vi "FCI Bin Test_102.vi"(8 "Error In":errorcluster, 9 "Calibration Image in":T1, 10 "Measurement Values array in":dbl[](array[numeric]), 11 "Image In":T1) -> (0 "Error Out":errorcluster, 1 "Measurement Values array out":dbl[](array[numeric]), 2 "102 Results":T2, 3 "Image Out":T1(plugin-control))   [LabVIEW 2019, in "Algorithm.lvclass"]
uses:
  FrameworkOverrides/Algorithm.lvclass
  <vilib>/vision/Image Controls.llb/IMAQ Image.ctl
panel:
  out "Algo Execution Time":u64
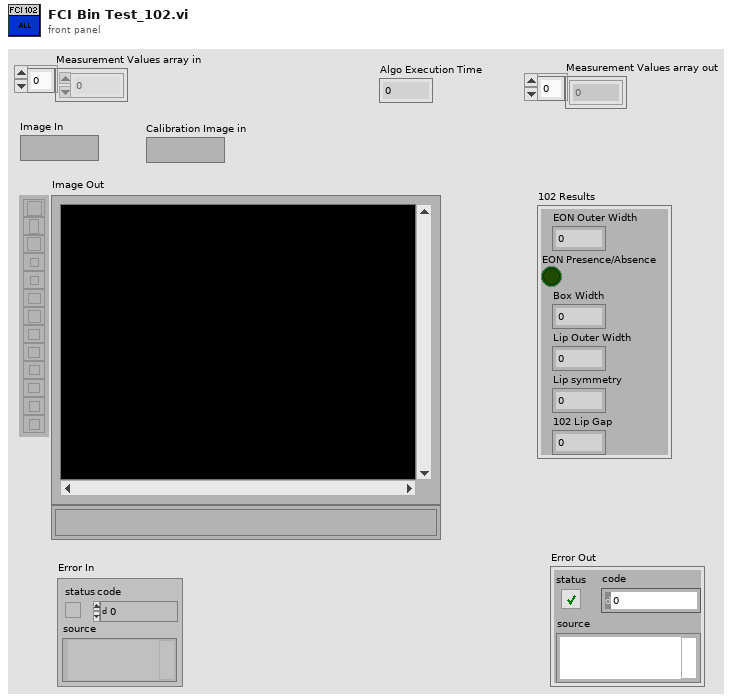
[diagram p1: front panel]
types:
  T1 = typedef "IMAQ Image.ctl" = refnum<image>
  T2 = cluster{"EON Outer Width":sgl, "EON Presence/Absence":bool, "Box Width":sgl, "Lip Outer Width":sgl, "Lip symmetry":dbl, "102 Lip Gap":sgl}
  T3 = cluster{"Box Width M ROI":cluster{"Left":dbl, "Top":dbl, "Right":dbl, "Bottom":dbl, "Angle":dbl}, "EON Outer Width M ROI":cluster{"Left":dbl, "Top":dbl, "Right":dbl, "Bottom":dbl, "Angle":dbl}, "Lip Outer Width M ROI":cluster{"Left":dbl, "Top":dbl, "Right":dbl, "Bottom":dbl, "Angle":dbl}, "102 Lip Gap M ROI":cluster{"Left":dbl, "Top":dbl, "Right":dbl, "Bottom":dbl, "Angle":dbl}}
  T4 = cluster{"Left":dbl, "Top":dbl, "Right":dbl, "Bottom":dbl, "Angle":dbl}
  T5 = typedef "Image Type" = u32
  T6 = cluster{"Centre X":dbl, "Centre Y":dbl, "Angle":dbl}
  T7 = cluster{"First Edges":cluster{"X":sgl, "Y":sgl}[], "Last Edges":cluster{"X":sgl, "Y":sgl}[]}
  T8 = cluster{cluster{"X":sgl, "Y":sgl}, cluster{"X":sgl, "Y":sgl}}[]
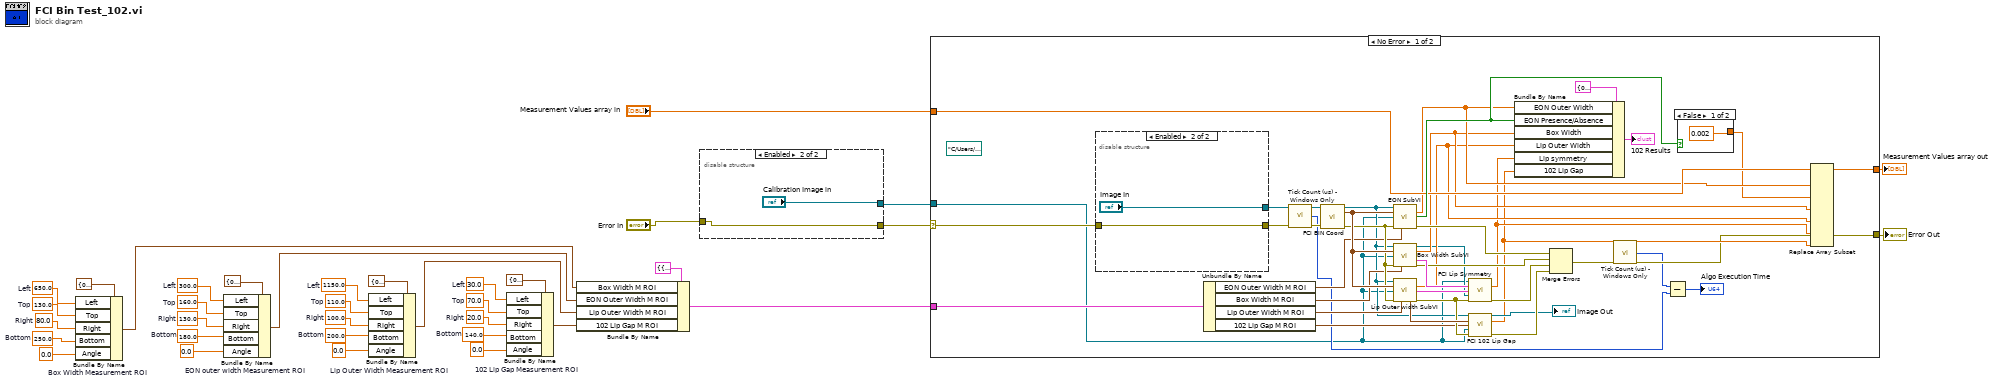
[diagram p0: block diagram]
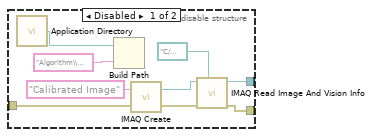
[diagram p2: hidden frame]
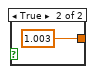
[diagram p3: hidden frame]
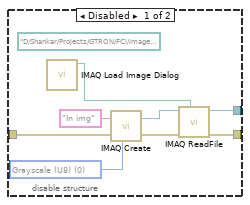
[diagram p4: hidden frame]
diagram:
  w27 = 140.0  # Bottom
  w28 = 20.0  # Right
  w29 = 70.0  # Top
  w30 = 30.0  # Left
  w21 = 200.0  # Bottom
  w20 = 100.0  # Right
  w19 = 110.0  # Top
  w18 = 1150.0  # Left
  w16 = 180.0  # Bottom
  w15 = 130.0  # Right
  w14 = 160.0  # Top
  w13 = 300.0  # Left
  w10 = 250.0  # Bottom
  w9 = 80.0  # Right
  w8 = 130.0  # Top
  w7 = 650.0  # Left
  n1 = Bundle By Name "Box Width Measurement ROI"(cluster=T4 {"Left"=0.0, "Top"=0.0, "Right"=0.0, "Bottom"=0.0, "Angle"=0.0} ("input cluster"), "Left"=w7, "Top"=w8, "Right"=w9, "Bottom"=w10, "Angle"=0.0) -> (w32:T4)
  n2 = Bundle By Name "EON outer width Measurement ROI"(cluster=T4 {"Left"=0.0, "Top"=0.0, "Right"=0.0, "Bottom"=0.0, "Angle"=0.0} ("input cluster"), "Left"=w13, "Top"=w14, "Right"=w15, "Bottom"=w16, "Angle"=0.0) -> (w33:T4)
  n3 = Bundle By Name "Lip Outer Width Measurement ROI"(cluster=T4 {"Left"=0.0, "Top"=0.0, "Right"=0.0, "Bottom"=0.0, "Angle"=0.0} ("input cluster"), "Left"=w18, "Top"=w19, "Right"=w20, "Bottom"=w21, "Angle"=0.0) -> (w34:T4)
  n4 = Bundle By Name "102 Lip Gap Measurement ROI"(cluster=T4 {"Left"=0.0, "Top"=0.0, "Right"=0.0, "Bottom"=0.0, "Angle"=0.0} ("input cluster"), "Left"=w30, "Top"=w29, "Right"=w28, "Bottom"=w27, "Angle"=0.0) -> (w35:T4)
  n5 = Bundle By Name(cluster=T3 {"Box Width M ROI"={"Left"=0.0, "Top"=0.0, "Right"=0.0, "Bottom"=0.0, "Angle"=0.0}, "EON Outer Width M ROI"={"Left"=0.0, "Top"=0.0, "Right"=0.0, "Bottom"=0.0, "Angle"=0.0}, "Lip Outer Width M ROI"={"Left"=0.0, "Top"=0.0, "Right"=0.0, "Bottom"=0.0, "Angle"=0.0}, "102 Lip Gap M ROI"={"Left"=0.0, "Top"=0.0, "Right"=0.0, "Bottom"=0.0, "Angle"=0.0}} ("output cluster"), "Box Width M ROI"=w32, "EON Outer Width M ROI"=w33, "Lip Outer Width M ROI"=w34, "102 Lip Gap M ROI"=w35) -> (w6:T3)
  n6 = disable-structure shown="Enabled" {
    disable-tunnel: "Error In" -> [w41 w47]
    disable-tunnel: [w39 w47] -> w2
    disable-tunnel: [w38 "Calibration Image in"] -> w1
    frame Disabled {
      n7 = call <vilib>:"Application Directory.vi"() -> ("Application Directory"=w45:path)
      n8 = Build Path(base path=w45, name or relative path="Algorithm\\calib images\\TL Calibrated Image.png") -> ()  [unwired: 1 out]
      n9 = call "IMAQ Create"("Image Name"="Calibrated Image", "error in (no error)"=w41) -> ("New Image"=w42:T1, "error out"=w40:errorcluster)  [unwired: 3 in]
      n10 = call "IMAQ Read Image And Vision Info"("File Path"=path "C:/Users/zentron/Desktop/Zengage/102 updated/Zengage 1.0/Algorithm/calib images/TL Calibrated Image.png", "error in (no error)"=w40, "Image"=w42) -> ("error out"=w39:errorcluster, "Image Out"=w38:T1)  [unwired: 6 in, 1 out]
    }
    frame Enabled {
    }
  }
  n11 = case shown="No Error" w2 {
    selector: w2 -> [w84 w100]
    tunnel: [w52 w100] -> w36
    tunnel: w6 -> [w74 _]
    tunnel: "Measurement Values array in" -> [w65 w99]
    tunnel: [w58 w99] -> w4
    tunnel: w1 -> [w48 _]
    frame No Error {
      (unwired) path "C:/Users/raakeshs/Desktop/LabVIEW Codes/GTRON Versions/Algo Test Code/Zengage 1.0/Algorithm/calib images/TL Calibrated Image.png" ("File Path")
      n12 = disable-structure shown="Enabled" {
        disable-tunnel: [w92 w98] -> w55
        disable-tunnel: w84 -> [w91 w98]
        disable-tunnel: [w90 "Image In"] -> w85
        frame Disabled {
          (unwired) path "D:/Shankar/Projects/GTRON/FCI/Images/FCI Img/102/Top Left/102_2_TL.png" ("Path")
          w94 = T5 0 items=["Grayscale (U8)", "Grayscale (I16)", "Grayscale (SGL)", "Complex (CSG)", "RGB (U32)", "HSL (U32)", "RGB (U64)", "Grayscale (U16)"] ("Image Type")
          n13 = call "IMAQ Load Image Dialog"() -> ("Path"=w89:path)  [unwired: 9 in, 2 out]
          n14 = call "IMAQ Create"("Image Name"="In img", "Image Type"=w94, "error in (no error)"=w91) -> ("New Image"=w96:T1, "error out"=w93:errorcluster)  [unwired: 2 in]
          n15 = call "IMAQ ReadFile"("File Path"=w89, "error in (no error)"=w93, "Image"=w96) -> ("error out"=w92:errorcluster, "Image Out"=w90:T1)  [unwired: 4 in, 3 out]
        }
        frame Enabled {
        }
      }
      n16 = Unbundle By Name(w74) -> ("EON Outer Width M ROI"=w73:T4, "Box Width M ROI"=w72:T4, "Lip Outer Width M ROI"=w71:T4, "102 Lip Gap M ROI"=w70:T4)
      n17 = call "Tick Count (us) - Windows Only.vi"("error in (no error)"=w55) -> ("micorsecond timer value"=w50:u64, "error out"=w54:errorcluster)  [unwired: 13 in]
      n18 = call "FCI BIN Coord.vi"("Image In"=w85, "error in (no error)"=w54) -> ("Image Out"=w57:T1, "Coord details"=w86:T6, "error IO"=w80:errorcluster)  [unwired: 11 in]
      n19 = call "EON SubVI.vi"("Image"=w57, "Coord details"=w86, "Calibrated Image"=w48, "error in (no error)"=w80, "M ROI"=w73) -> ("EON outer width"=w64:sgl, "EON Presence/Absence"=w66:bool, "error out"=w78:errorcluster)  [unwired: 7 in, 1 out]
      n20 = call "Box Width SubVI.vi"("Image"=w57, "Coord details"=w86, "Calibrated Image"=w48, "error in (no error)"=w80, "M ROI"=w72) -> ("Image Out"=w56:T1, "Box Width"=w62:sgl, "All Edges"=w83:T7, "error out"=w77:errorcluster)  [unwired: 7 in]
      n21 = call "Lip Outer width SubVI.vi"("Image"=w57, "Coord details"=w86, "Calibrated Image"=w48, "error in (no error)"=w80, "M ROI"=w71) -> ("Lip Outer Width"=w61:sgl, "Perpendicular Lines"=w82:T8, "Edge Coordinates"=w81:cluster{"X":sgl, "Y":sgl}[], "error out"=w79:errorcluster)  [unwired: 6 in, 1 out]
      n22 = call "FCI Lip Symmetry.vi"("Calibrated Image"=w48, "Box All Edges"=w83, "Lip Outer Perpendicular lines"=w82, "Image in"=w56, "error in (no error)"=w79) -> ("Lip symmetry"=w60:dbl, "error out"=w76:errorcluster)  [unwired: 9 in]
      n23 = call "FCI 102 Lip Gap.vi"("Image"=w57, "Lip Outer Points"=w81, "M ROI"=w70, "Calibrated Image"=w48, "error in (no error)"=w79) -> ("Image Out"=→"Image Out":T1, "102 Lip Gap"=w59:sgl, "error out"=w75:errorcluster)  [unwired: 8 in]
      n24 = Bundle By Name(cluster=T2 {"EON Outer Width"=0.0, "EON Presence/Absence"=FALSE, "Box Width"=0.0, "Lip Outer Width"=0.0, "Lip symmetry"=0.0, "102 Lip Gap"=0.0} ("output cluster"), "EON Outer Width"=w64, "EON Presence/Absence"=w66, "Box Width"=w62, "Lip Outer Width"=w61, "Lip symmetry"=w60, "102 Lip Gap"=w59) -> (→"102 Results":T2)
      n25 = Merge Errors(w78, w77, w76, w75) -> (w53:errorcluster)
      n26 = call "Tick Count (us) - Windows Only.vi"("error in (no error)"=w53) -> ("micorsecond timer value"=w51:u64, "error out"=w52:errorcluster)  [unwired: 13 in]
      n27 = Subtract(x=w51, y=w50) -> (x-y=→"Algo Execution Time":u64)
      n28 = case shown="False" w66 {
        tunnel: [0.002 1.003] -> w63
        frame False {
        }
        frame True {
        }
      }
      n29 = Replace Array Subset(array=w65, new element #1=w64, new element #2=w63, new element #3=w62, new element #4=w61, new element #5=w60, new element #6=w59) -> (w58:dbl[])  [unwired: 6 in]
    }
    frame Error {
    }
  }
  "Error Out" <- w36
  "Measurement Values array out" <- w4
